vi "ORS_GalvoPrepareScan_uw-1kp.vi"(7 "SampQuant.SampMode":i32(ring)=10123 items=["Finite Samples"=10178, "Continuous Samples"=10123, "Hardware Timed Single Point"=12522], 8 "error in":errorcluster, 9 "use_digi_trig":bool, 10 "AO.DataXferMech":i32(ring)=12590 items=["DMA"=10054, "Interrupts"=10204, "Programmed I/O"=10264, "USB Bulk"=12590], 11 "Galvo":T1={"x mirror"="Dev1/ao0", "y mirror"="Dev1/ao1", "trig out"="Dev1/port0/line2", "x mirror task"="", "y mirror task"="", "trig out task"="", "n_axis"=0, "params"={"n_lines"=500, "n_frames"=400, "force to zero"=FALSE, "Triggers_per_sweep"=1.0, "X center"=0.0, "X span"=3.4000000000000004, "Y center"=0.0, "Y span"=0.0, "flyb.lines"=40, "n_triggers"=1, "mode"=3, "offset"=0.0, "galvo phase"=0, "span factor"=0.0, "Custom trig."={"n_f to c. trig"=0, "c. trig length"=0, "c. trig interval"=0, "n_c. trig"=0}, "f_per_pos"=1, "n_dataset"=1, "flyback fr"=0}, "acq trig out"="Dev1/port0/line4", "acq trig out task"="", "sample array X"=[], "sample array Y"=[], "custom trig out"="", "custom trig out task"="", "FDML-box"="TCPIP0::10.153.218.51::23::SOCKET", "ACQ/Galvo"=enum."NI_DAQ", "acq trig out an task"="", "acq trig out an"="Dev1/ao2", "Galvo Trig input"="/Dev1/PFI1", "Galvo Clk input"="OnboardClock", "sample array Acq trig out an"=[]} {"params"."n_dataset" min=1; "params"."X center" format="%^_3g"; "params"."X span" format="%^_3g"; "params"."Y center" format="%^_3g"; "params"."Y span" format="%^_3g"}) -> (0 "error out":errorcluster, 1 "# samples":i32, 2 "Galvo wfm":dbl[][](graph), 3 "Galvo out":T1={"x mirror"="Dev1/ao0", "y mirror"="Dev1/ao1", "trig out"="Dev1/port0/line2", "x mirror task"="", "y mirror task"="", "trig out task"="", "n_axis"=0, "params"={"n_lines"=500, "n_frames"=400, "force to zero"=FALSE, "Triggers_per_sweep"=1.0, "X center"=0.0, "X span"=3.4000000000000004, "Y center"=0.0, "Y span"=0.0, "flyb.lines"=40, "n_triggers"=1, "mode"=3, "offset"=0.0, "galvo phase"=0, "span factor"=0.0, "Custom trig."={"n_f to c. trig"=0, "c. trig length"=0, "c. trig interval"=0, "n_c. trig"=0}, "f_per_pos"=1, "n_dataset"=1, "flyback fr"=0}, "acq trig out"="Dev1/port0/line4", "acq trig out task"="", "sample array X"=[], "sample array Y"=[], "custom trig out"="", "custom trig out task"="", "FDML-box"="TCPIP0::10.153.218.51::23::SOCKET", "ACQ/Galvo"=enum."NI_DAQ", "acq trig out an task"="", "acq trig out an"="Dev1/ao2", "Galvo Trig input"="/Dev1/PFI1", "Galvo Clk input"="OnboardClock", "sample array Acq trig out an"=[]} {"params"."n_dataset" min=1; "params"."X center" format="%^_3g"; "params"."X span" format="%^_3g"; "params"."Y center" format="%^_3g"; "params"."Y span" format="%^_3g"})   [LabVIEW 2024]
uses:
  Typedefs/ORS_Galvo.ctl
  Typedefs/ORS_Galvo_params.ctl
  <vilib>/Utility/error.llb/DialogType.ctl
  <vilib>/DAQmx/write.llb/DAQmx Write (Digital Bool 1Line 1Point).vi
  <vilib>/DAQmx/write.llb/DAQmx Write (Analog DBL 1Chan 1Samp).vi
  <vilib>/DAQmx/write.llb/DAQmx Write (Analog 2D DBL NChan NSamp).vi
  <vilib>/DAQmx/write.llb/DAQmx Write (Analog 1D DBL NChan 1Samp).vi
  <vilib>/DAQmx/write.llb/DAQmx Write (Digital 2D U32 NChan NSamp).vi
  <vilib>/DAQmx/write.llb/DAQmx Write (Analog 1D DBL 1Chan NSamp).vi
  <vilib>/DAQmx/miscellaneous.llb/DAQmx Fill In Error Info.vi
  <resource>/objmgr/daqmx.rc
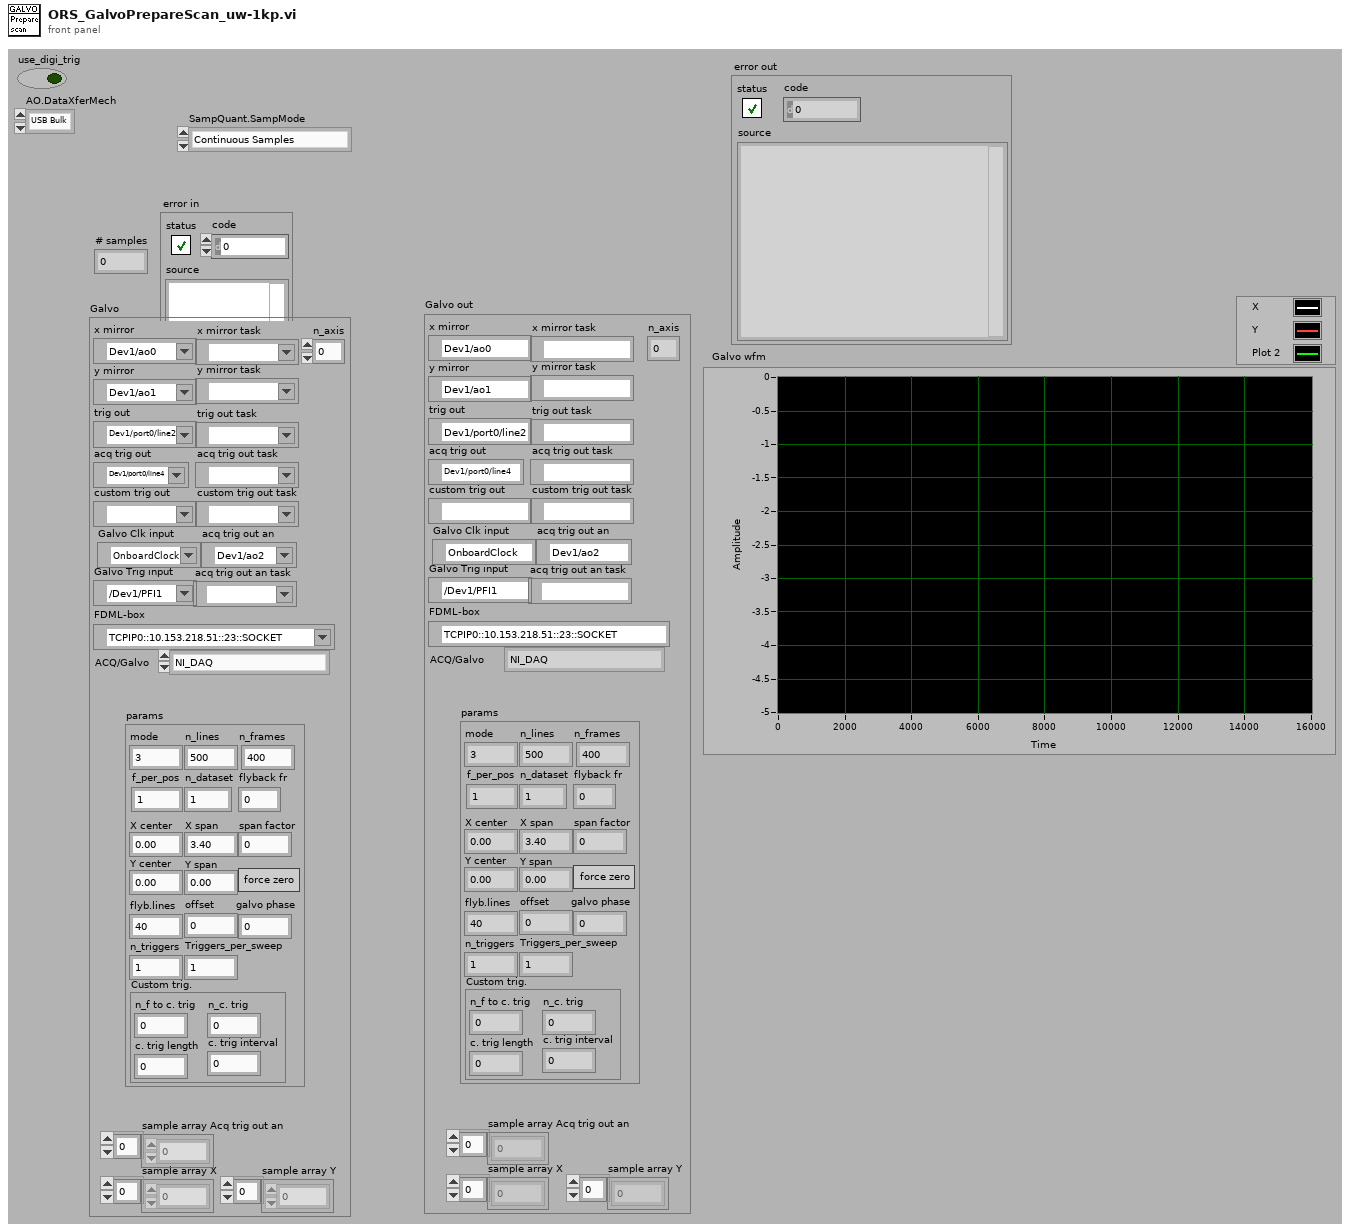
[diagram p1: front panel]
types:
  T1 = typedef "ORS_Galvo.ctl" = cluster{"x mirror":tag, "y mirror":tag, "trig out":tag, "x mirror task":refnum<k21>, "y mirror task":refnum<k21>, "trig out task":refnum<k21>, "n_axis":i32, "params":T2, "acq trig out":tag, "acq trig out task":refnum<k21>, "sample array X":dbl[], "sample array Y":dbl[], "custom trig out":tag, "custom trig out task":refnum<k21>, "FDML-box":refnum<visa-resource-name>, "ACQ/Galvo":enum16{"ADC/FDML", "NI_DAQ", "ADC"}, "acq trig out an task":refnum<k21>, "acq trig out an":tag, "Galvo Trig input":tag, "Galvo Clk input":tag, "sample array Acq trig out an":dbl[]}
  T2 = typedef "ORS_Galvo_params.ctl" = cluster{"n_lines":i32, "n_frames":i32, "force to zero":bool, "Triggers_per_sweep":dbl, "X center":dbl, "X span":dbl, "Y center":dbl, "Y span":dbl, "flyb.lines":i32, "n_triggers":i32, "mode":i32, "offset":dbl, "galvo phase":i32, "span factor":dbl, "Custom trig.":cluster{"n_f to c. trig":i32, "c. trig length":i32, "c. trig interval":i32, "n_c. trig":i32}, "f_per_pos":i32, "n_dataset":u32, "flyback fr":u16}
  T3 = typedef "DialogType.ctl" = u16
  T4 = cluster{"n_f to c. trig":i32, "c. trig length":i32, "c. trig interval":i32, "n_c. trig":i32}
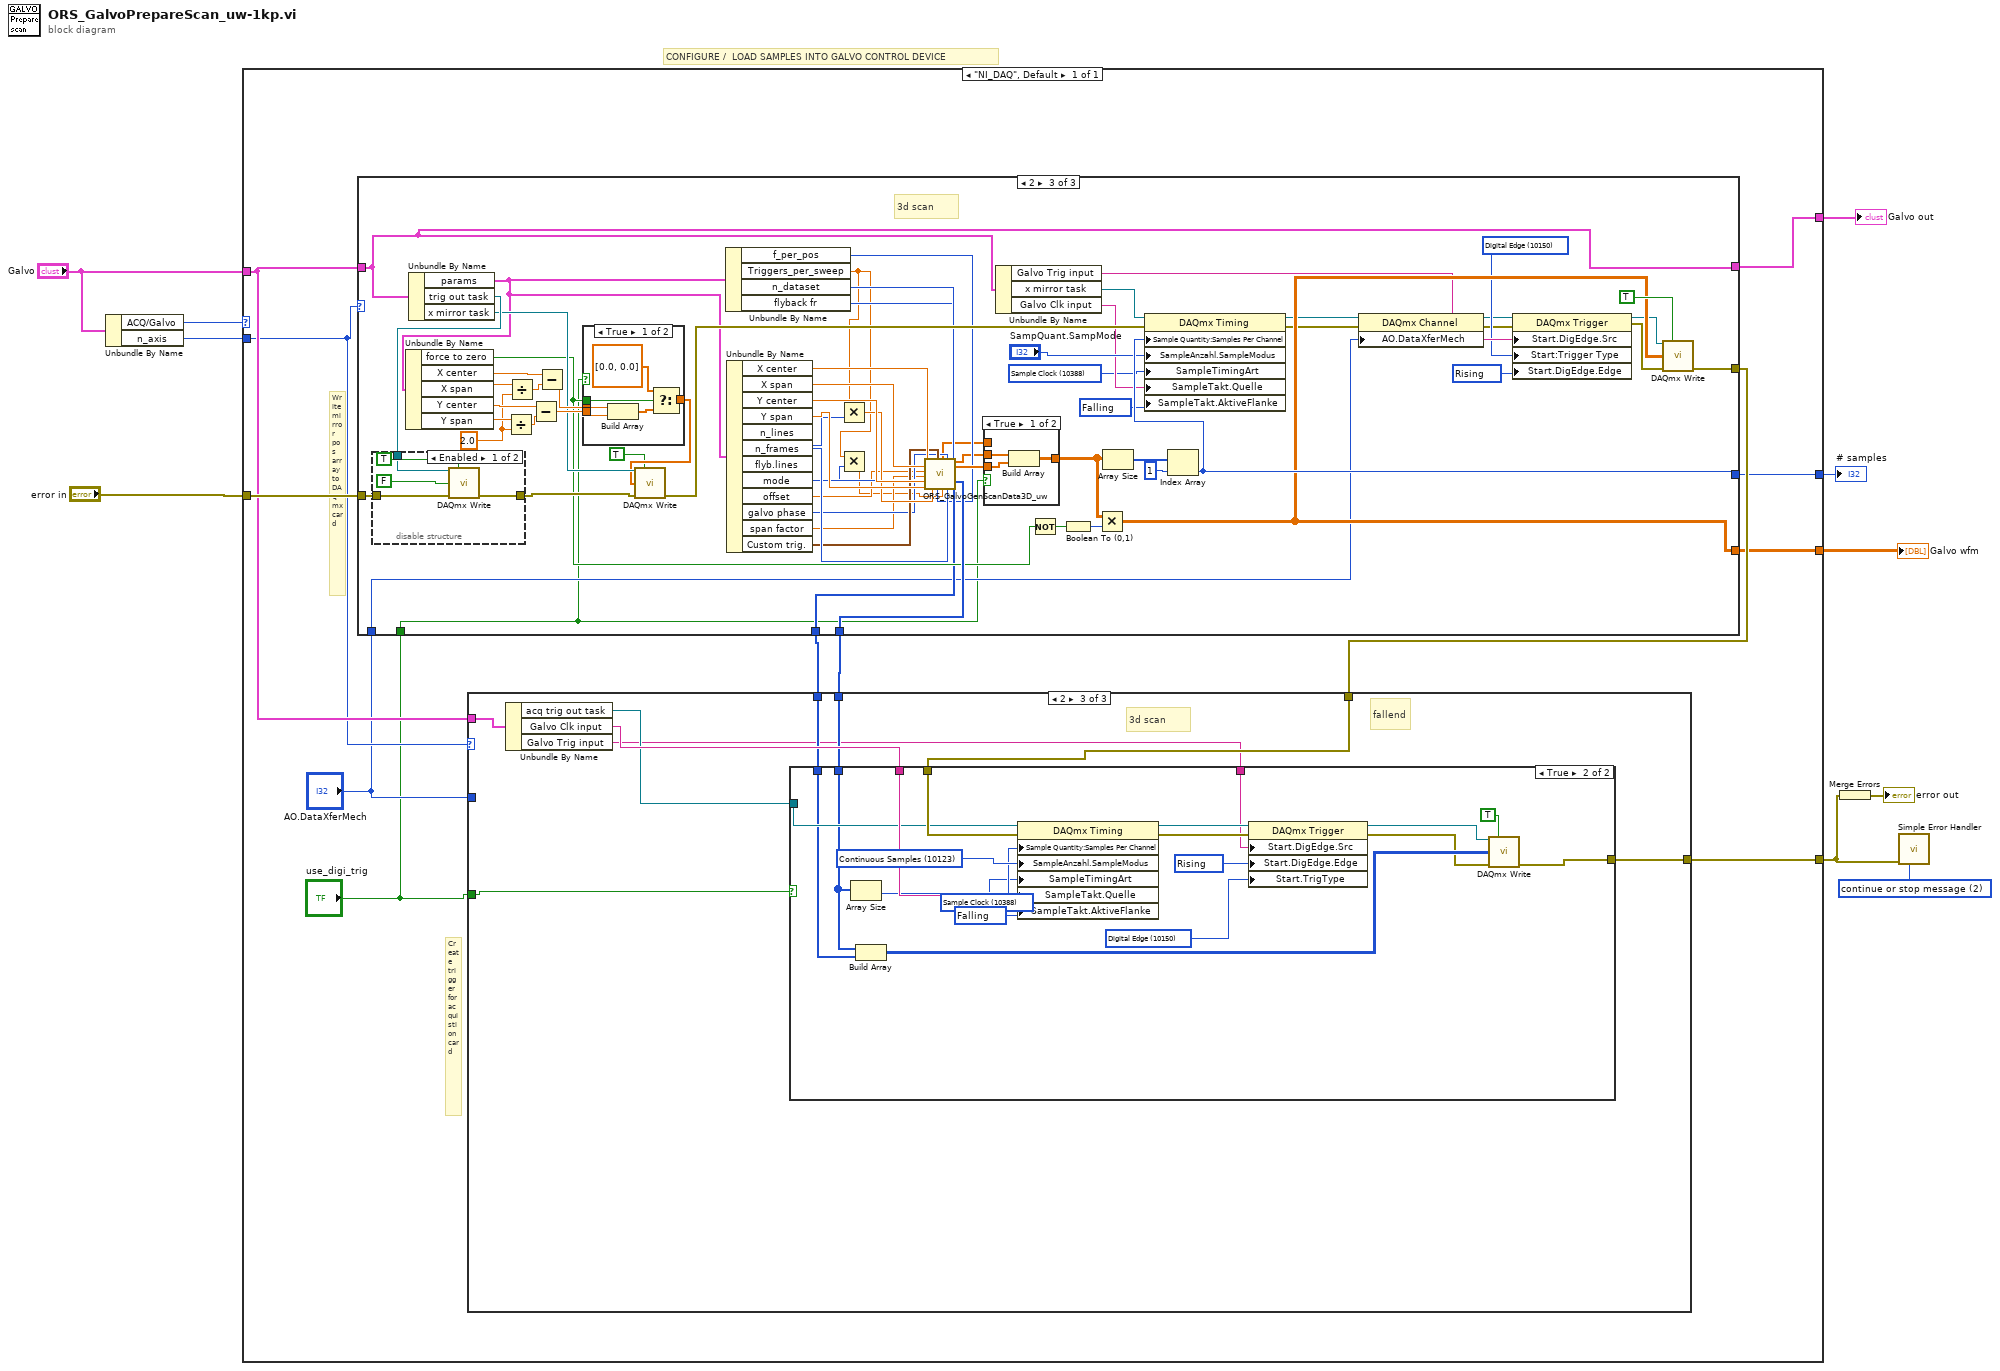
[diagram p0: block diagram]
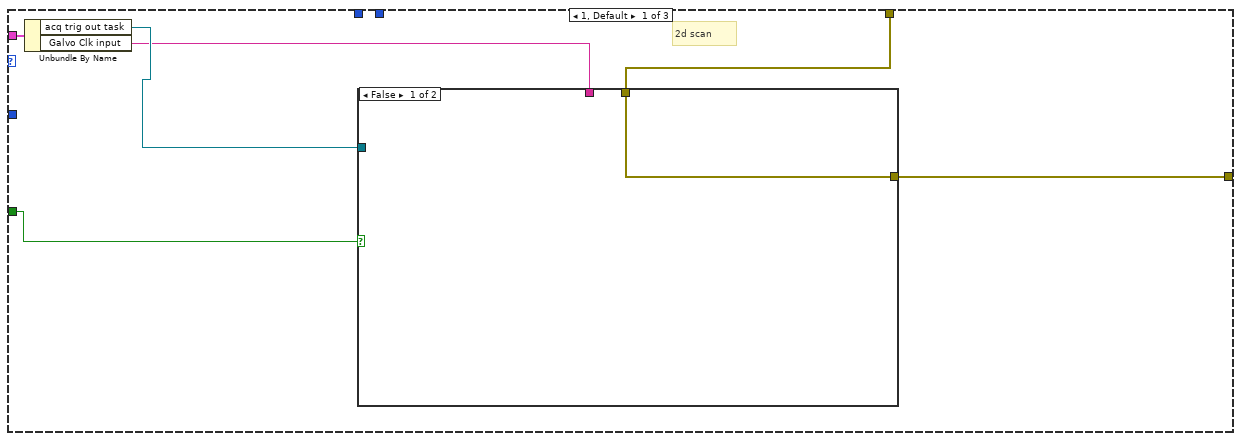
[diagram p2: hidden frame]
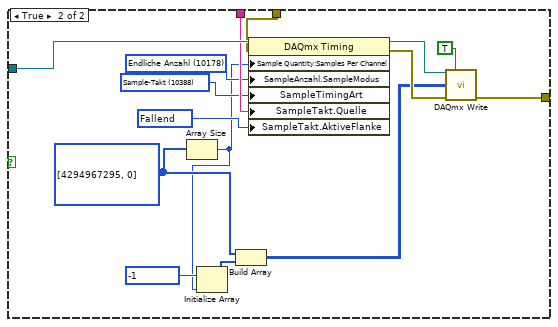
[diagram p3: hidden frame]
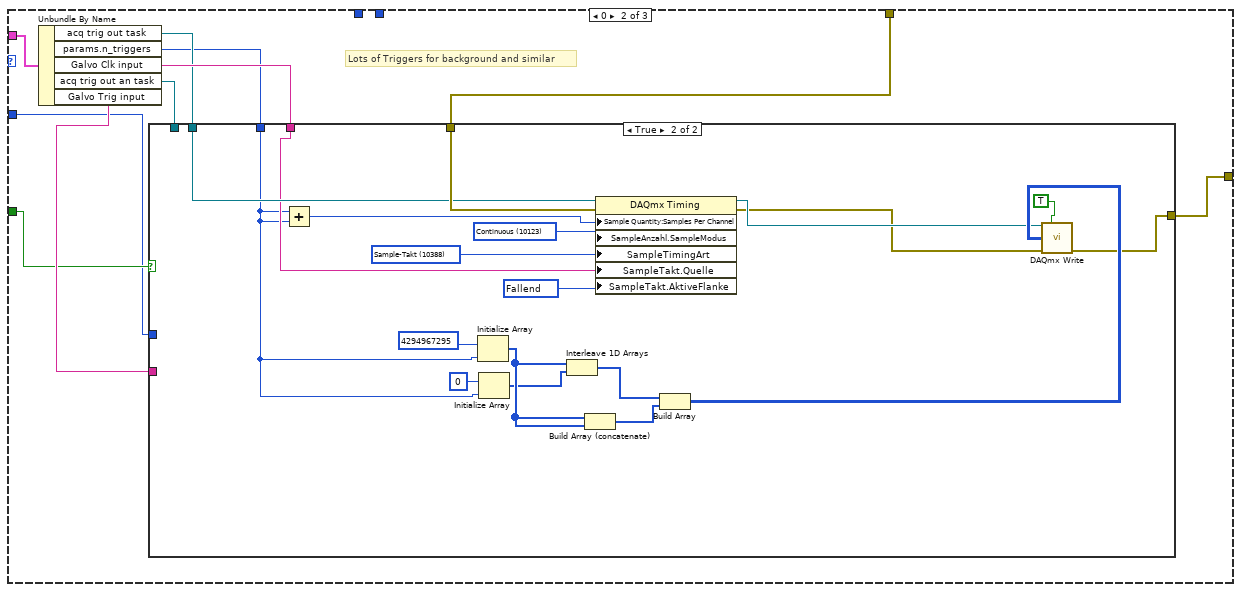
[diagram p4: hidden frame]
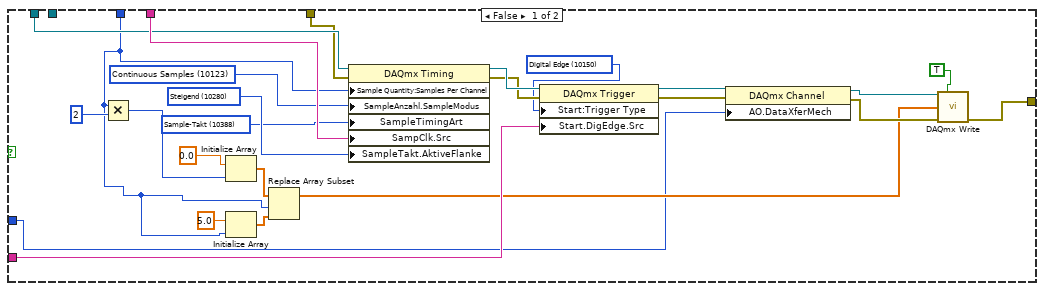
[diagram p5: hidden frame]
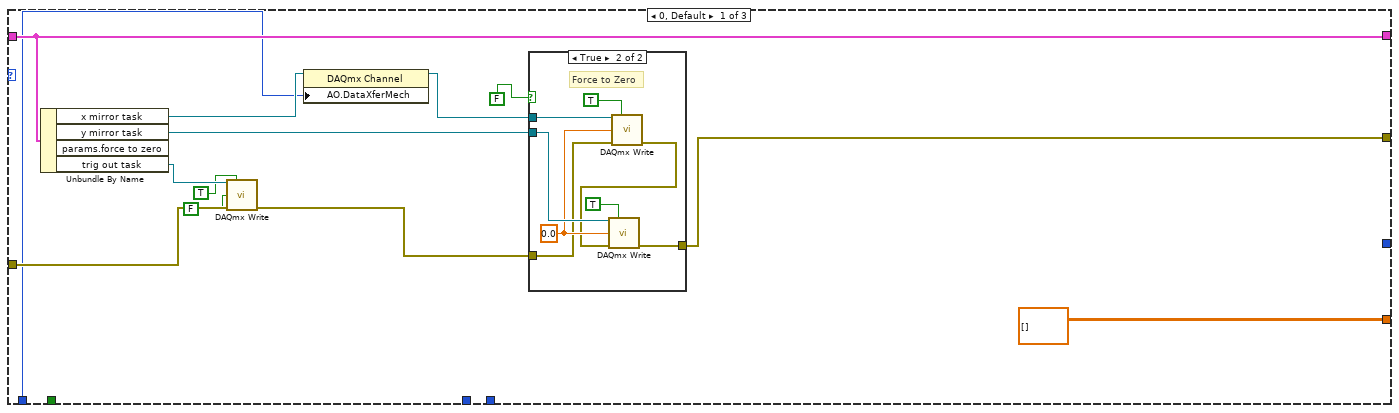
[diagram p7: hidden frame]
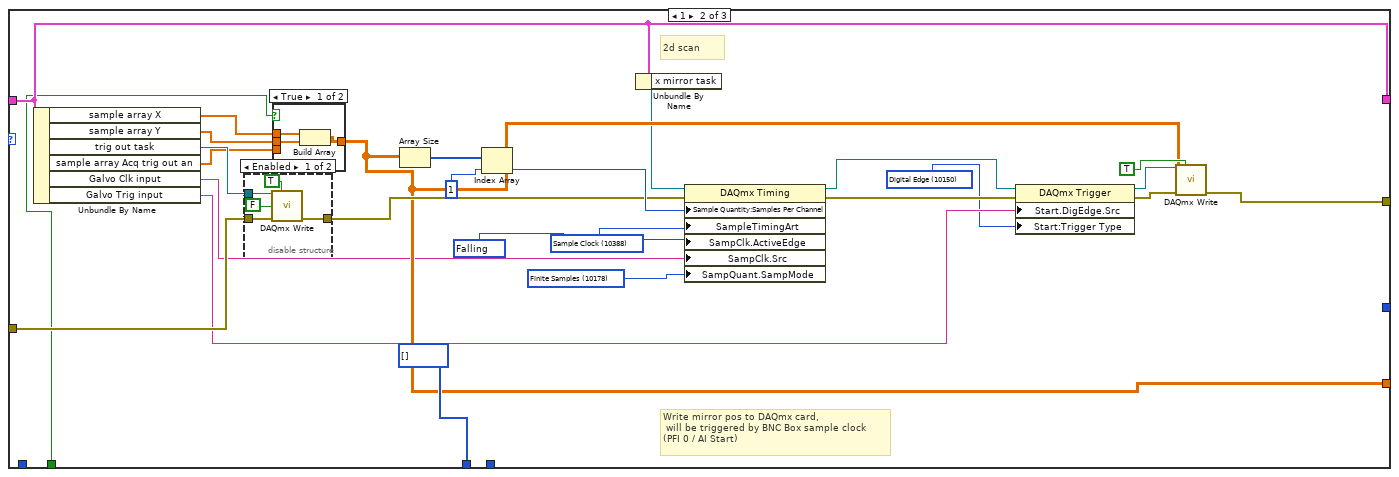
[diagram p9: hidden frame]
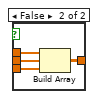
[diagram p11: hidden frame]
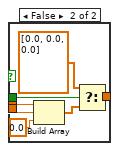
[diagram p13: hidden frame]
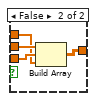
[diagram p14: hidden frame]
diagram:
  w7 = T3 2 items=["no dialog", "OK message", "continue or stop message", "OK message + warnings", "continue/stop + warnings"] ("type of dialog (OK msg:1)")
  # "CONFIGURE /  LOAD SAMPLES INTO GALVO CONTROL DEVICE"
  n1 = Unbundle By Name("Galvo") -> ("ACQ/Galvo"=w2:enum16{"ADC/FDML", "NI_DAQ", "ADC"}, "n_axis"=w1:i32)
  n2 = case shown="\"NI_DAQ\", Default" w2 {
    tunnel: "error in" -> [w22]
    tunnel: [w20] -> w8
    tunnel: [w17] -> w6
    tunnel: "Galvo" -> [w16]
    tunnel: [w15] -> w5
    tunnel: [w14] -> w4
    tunnel: w1 -> [w13]
    frame "NI_DAQ", Default {
      # "Write mirror pos array to DAQmx card"
      # "Create trigger for acquistion card"
      n3 = case shown="2" w13 {
        tunnel: w22 -> [w136 w174 w243]
        tunnel: [w139 w172 w252] -> w21
        tunnel: [w140 w161 w250] -> w17
        tunnel: w16 -> [w140 w161 w250]
        tunnel: [_ _ w244] -> w19
        tunnel: [_ u32[] [] ("custom trig out") w221] -> w18
        tunnel: [_ _ w212] -> w15
        tunnel: [dbl[][] [] w163 w206] -> w14
        tunnel: "AO.DataXferMech" -> [w128 _ w192]
        tunnel: "use_digi_trig" -> [_ w150 w191]
        frame 0, Default {
          n4 = Unbundle By Name(w140) -> ("x mirror task"=w132:refnum<k21>, "y mirror task"=w138:refnum<k21>, "trig out task"=w137:refnum<k21>)  [unwired: 1 out]
          n5 = call-poly <vilib>:"DAQmx Write.vi"("task/channels in"=w137, "auto start"=TRUE, "data"=FALSE, "error in"=w136) -> ("error out"=w135:errorcluster)  [unwired: 9 in, 2 out]
          n6 = property class="DAQmx Channel"(reference=w132, "AO.DataXferMech"=w128) -> (reference out=w131:refnum<k21>)  [unwired: 1 in, 1 out]
          n7 = case shown="True" FALSE {
            tunnel: w138 -> [_ w149]
            tunnel: w135 -> [w141 w143]
            tunnel: [w141 w147] -> w139
            tunnel: w131 -> [_ w145]
            frame False {
            }
            frame True {
              w144 = 0.0 ("t")
              # "Force to Zero"
              n8 = call-poly <vilib>:"DAQmx Write.vi"("task/channels in"=w145, "auto start"=TRUE, "data"=w144, "error in"=w143) -> ("error out"=w142:errorcluster)  [unwired: 9 in, 2 out]
              n9 = call-poly <vilib>:"DAQmx Write.vi"("task/channels in"=w149, "auto start"=TRUE, "data"=w144, "error in"=w142) -> ("error out"=w147:errorcluster)  [unwired: 9 in, 2 out]
            }
          }
        }
        frame 1 {
          w151 = 10150 items=["Analog Edge"=10099, "Digital Edge"=10150, "Digital Pattern"=10398, "Analog Window"=10103, "None"=10230] ("Start.TrigType")
          w158 = 10178 items=["Finite Samples"=10178, "Continuous Samples"=10123, "Hardware Timed Single Point"=12522] ("SampQuant.SampMode")
          w159 = 10388 items=["Sample Clock"=10388, "Burst Handshake"=12548, "Handshake"=10389, "Implicit"=10451, "On Demand"=10390, "Change Detection"=12504, "Pipelined Sample Clock"=14668] ("SampTimingType")
          w164 = 10171 items=["Rising"=10280, "Falling"=10171] ("SampClk.ActiveEdge")
          # "2d scan"
          # "Write mirror pos to DAQmx card,\n will be triggered by BNC Box sample clock\n(PFI 0 / AI Start)"
          n10 = Unbundle By Name(w161) -> ("sample array X"=w171:dbl[], "sample array Y"=w170:dbl[], "trig out task"=w175:refnum<k21>, "sample array Acq trig out an"=w162:dbl[], "Galvo Clk input"=w153:tag, "Galvo Trig input"=w154:tag)
          n11 = disable-structure shown="Enabled" {
            disable-tunnel: w175 -> [w180 _]
            disable-tunnel: w174 -> [w178 w181]
            disable-tunnel: [w176 w181] -> w166
            frame Enabled {
              n12 = call-poly <vilib>:"DAQmx Write.vi"("task/channels in"=w180, "auto start"=TRUE, "data"=FALSE, "error in"=w178) -> ("error out"=w176:errorcluster)  [unwired: 9 in, 2 out]
            }
            frame Disabled {
            }
          }
          n13 = case shown="True" w150 {
            tunnel: w171 -> [w184 w188]
            tunnel: w170 -> [w183 w187]
            tunnel: [w182 w186] -> w163
            tunnel: w162 -> [_ w185]
            frame True {
              n14 = Build Array(w184, w183) -> (w182:dbl[][])
            }
            frame False {
              n15 = Build Array(w188, w187, w185) -> (w186:dbl[][])
            }
          }
          n16 = Array Size(array=w163) -> (size(s)=w169:i32[])
          n17 = Index Array(array=w169, index=1) -> (element=w167:i32)
          n18 = Unbundle By Name(w161) -> ("x mirror task"=w160:refnum<k21>)
          n19 = property class="DAQmx Timing"(reference=w160, error in=w166, "Sample Quantity:Samples Per Channel"=w167, "SampleTimingArt"=w159, "SampClk.ActiveEdge"=w164, "SampClk.Src"=w153, "SampQuant.SampMode"=w158) -> (reference out=w152:refnum<k21>, error out=w156:errorcluster)
          n20 = property class="DAQmx Trigger"(reference=w152, error in=w156, "Start.DigEdge.Src"=w154, "Start:Trigger Type"=w151) -> (reference out=w157:refnum<k21>, error out=w155:errorcluster)
          n21 = call-poly <vilib>:"DAQmx Write.vi"("task/channels in"=w157, "auto start"=TRUE, "data"=w163, "error in"=w155) -> ("error out"=w172:errorcluster)  [unwired: 9 in, 2 out]
        }
        frame 2 {
          w189 = 10171 items=["Rising"=10280, "Falling"=10171] ("SampClk.ActiveEdge")
          w190 = 10388 items=["Sample Clock"=10388, "Burst Handshake"=12548, "Handshake"=10389, "Implicit"=10451, "On Demand"=10390, "Change Detection"=12504, "Pipelined Sample Clock"=14668] ("SampTimingType")
          w193 = 10280 items=["Rising"=10280, "Falling"=10171] ("Start.DigEdge.Edge")
          w199 = 10150 items=["Analog Edge"=10099, "Digital Edge"=10150, "Digital Pattern"=10398, "Analog Window"=10103, "None"=10230] ("Start.TrigType")
          w230 = 2.0
          # "3d scan"
          n22 = Unbundle By Name(w250) -> ("params"=w224:T2, "trig out task"=w242:refnum<k21>, "x mirror task"=w235:refnum<k21>)
          n23 = disable-structure shown="Enabled" {
            disable-tunnel: w243 -> [w258 w261]
            disable-tunnel: w242 -> [w257 _]
            disable-tunnel: [w256 w261] -> w241
            frame Enabled {
              n24 = call-poly <vilib>:"DAQmx Write.vi"("task/channels in"=w257, "auto start"=TRUE, "data"=FALSE, "error in"=w258) -> ("error out"=w256:errorcluster)  [unwired: 9 in, 2 out]
            }
            frame Disabled {
            }
          }
          n25 = Unbundle By Name(w224) -> ("force to zero"=w225:bool, "X center"=w239:dbl, "X span"=w231:dbl, "Y center"=w238:dbl, "Y span"=w234:dbl)
          n26 = Divide(x=w234, y=w230) -> (x/y=w233:dbl)
          n27 = Divide(x=w231, y=w230) -> (x/y=w232:dbl)
          n28 = Subtract(x=w238, y=w233) -> (x-y=w236:dbl)
          n29 = Subtract(x=w239, y=w232) -> (x-y=w237:dbl)
          n30 = case shown="True" w191 {
            tunnel: w237 -> [w267 w274]
            tunnel: w236 -> [w266 w273]
            tunnel: [w264 w271] -> w229
            tunnel: w225 -> [w263 w270]
            frame True {
              n31 = Build Array(w267, w266) -> (w265:dbl[])
              n32 = Select(t=dbl[] [0.0, 0.0] ("s? t:f"), s=w263, f=w265) -> (s? t:f=w264:dbl[])
            }
            frame False {
              n33 = Build Array(w274, w273, 0.0 ("element")) -> (w272:dbl[])
              n34 = Select(t=dbl[] [0.0, 0.0, 0.0] ("s? t:f"), s=w270, f=w272) -> (s? t:f=w271:dbl[])
            }
          }
          n35 = call-poly <vilib>:"DAQmx Write.vi"("task/channels in"=w235, "auto start"=TRUE, "data"=w229, "error in"=w241) -> ("error out"=w240:errorcluster)  [unwired: 9 in, 2 out]
          n36 = Unbundle By Name(w224) -> ("f_per_pos"=w215:i32, "Triggers_per_sweep"=w210:dbl, "n_dataset"=w214:u32, "flyback fr"=w213:u16)
          n37 = Unbundle By Name(w224) -> ("X center"=w249:dbl, "X span"=w248:dbl, "Y center"=w247:dbl, "Y span"=w246:dbl, "n_lines"=w223:i32, "n_frames"=w245:i32, "flyb.lines"=w209:i32, "mode"=w219:i32, "offset"=w216:dbl, "galvo phase"=w218:i32, "span factor"=w217:dbl, "Custom trig."=w220:T4)
          n38 = Multiply(x=w210, y=w223) -> (x*y=w222:dbl)
          n39 = Multiply(x=w210, y=w209) -> (x*y=w208:dbl)
          n40 = call "ORS_GalvoGenScanData3D_uw.vi"("x_center"=w249, "x_span"=w248, "offset"=w216, "span-factor"=w217, "y_center"=w247, "y_span"=w246, "mode"=w219, "n_lines"=w222, "Custom trig."=w220, "n_frames same y pos"=w215, "flyback_lines"=w208, "galvo phase"=w218, "n_frames"=w245, "n_3D scans"=w214, "flyback frames"=w213) -> ("t_data"=w205:dbl[], "x_data"=w207:dbl[], "y_data"=w251:dbl[], "trigger out"=w244:u32[], "custom trig out"=w221:u32[])
          n41 = case shown="True" w191 {
            tunnel: w251 -> [w277 w281]
            tunnel: [w276 w280] -> w228
            tunnel: w207 -> [w275 w279]
            tunnel: w205 -> [_ w278]
            frame True {
              n42 = Build Array(w275, w277) -> (w276:dbl[][])
            }
            frame False {
              n43 = Build Array(w279, w281, w278) -> (w280:dbl[][])
            }
          }
          n44 = Unbundle By Name(w250) -> ("Galvo Trig input"=w202:tag, "x mirror task"=w253:refnum<k21>, "Galvo Clk input"=w200:tag)
          n45 = Not(x=w225) -> (.not. x?=w226:bool)
          n46 = Boolean To (0,1)(Boolean=w226) -> (0, 1=w227:i16)
          n47 = Multiply(x=w228, y=w227) -> (x*y=w206:dbl[][])
          n48 = Array Size(array=w228) -> (size(s)=w211:i32[])
          n49 = Index Array(array=w211, index=1 ("Index")) -> (element=w212:i32)
          n50 = property class="DAQmx Timing"(reference=w253, error in=w240, "Sample Quantity:Samples Per Channel"=w212, "SampleAnzahl.SampleModus"="SampQuant.SampMode", "SampleTimingArt"=w190, "SampleTakt.Quelle"=w200, "SampleTakt.AktiveFlanke"=w189) -> (reference out=w198:refnum<k21>, error out=w197:errorcluster)
          n51 = property class="DAQmx Channel"(reference=w198, error in=w197, "AO.DataXferMech"=w192) -> (reference out=w196:refnum<k21>, error out=w195:errorcluster)
          n52 = property class="DAQmx Trigger"(reference=w196, error in=w195, "Start.DigEdge.Src"=w202, "Start:Trigger Type"=w199, "Start.DigEdge.Edge"=w193) -> (reference out=w204:refnum<k21>, error out=w203:errorcluster)
          n53 = call-poly <vilib>:"DAQmx Write.vi"("task/channels in"=w204, "auto start"=TRUE, "data"=w206, "error in"=w203) -> ("error out"=w252:errorcluster)  [unwired: 9 in, 2 out]
        }
      }
      n54 = case shown="2" w13 {
        tunnel: w16 -> [w28 w54 w107]
        tunnel: [w24 w53 w104] -> w20
        tunnel: w21 -> [w26 w49 w106]
        tunnel: w19 -> [_ _ w101]
        tunnel: w18 -> [_ _ w102]
        tunnel: "use_digi_trig" -> [w23 w46 w100]
        tunnel: "AO.DataXferMech" -> [_ w45 _]
        frame 1, Default {
          # "2d scan"
          n55 = Unbundle By Name(w28) -> ("acq trig out task"=w27:refnum<k21>, "Galvo Clk input"=w25:tag)
          n56 = case shown="False" w23 {
            tunnel: w27 -> [_ w44]
            tunnel: w26 -> [w29 w43]
            tunnel: w25 -> [_ w42]
            tunnel: [w29 w41] -> w24
            frame False {
            }
            frame True {
              w34 = u32[] [4294967295, 0] ("data")
              w38 = 10171 items=["Steigend"=10280, "Fallend"=10171] ("SampleTakt.AktiveFlanke")
              w39 = 10178 items=["Endliche Anzahl"=10178, "kontinuierlich"=10123, "Einzelwert (HW-getaktet)"=12522] ("SampleAnzahl.SampleModus")
              w40 = 10388 items=["Sample-Takt"=10388, "Burst-Handshake"=12548, "Handshake"=10389, "implizit"=10451, "1 Sample"=10390, "Änderungserkennung"=12504, "Sample-Takt in Pipeline"=14668] ("SampleTimingArt")
              n57 = Array Size(array=w34) -> (size(s)=w31:i32)
              n58 = Initialize Array(-1 ("Waveform"), w31) -> (w30:i32[])
              n59 = Build Array(w34, w30) -> (w33:u32[][])
              n60 = property class="DAQmx Timing"(reference=w44, error in=w43, "Sample Quantity:Samples Per Channel"=w31, "SampleAnzahl.SampleModus"=w39, "SampleTimingArt"=w40, "SampleTakt.Quelle"=w42, "SampleTakt.AktiveFlanke"=w38) -> (reference out=w37:refnum<k21>, error out=w36:errorcluster)
              n61 = call-poly <vilib>:"DAQmx Write.vi"("task/channels in"=w37, "auto start"=TRUE, "data"=w33, "error in"=w36) -> ("error out"=w41:errorcluster)  [unwired: 9 in, 2 out]
            }
          }
        }
        frame 0 {
          # "Lots of Triggers for background and similar"
          n62 = Unbundle By Name(w54) -> ("acq trig out task"=w48:refnum<k21>, "params.n_triggers"=w47:i32, "Galvo Clk input"=w52:tag, "acq trig out an task"=w51:refnum<k21>, "Galvo Trig input"=w50:tag)
          n63 = case shown="True" w46 {
            tunnel: [w79 w84] -> w53
            tunnel: w52 -> [w78 w83]
            tunnel: w51 -> [w77 _]
            tunnel: w50 -> [w76 _]
            tunnel: w49 -> [w59 w86]
            tunnel: w48 -> [_ w85]
            tunnel: w47 -> [w56 w82]
            tunnel: w45 -> [w55 _]
            frame False {
              w60 = 10150 items=["Analog Edge"=10099, "Digital Edge"=10150, "Digital Pattern"=10398, "Analog Window"=10103, "None"=10230] ("Start.TrigType")
              w69 = 10123 items=["Finite Samples"=10178, "Continuous Samples"=10123, "Hardware Timed Single Point"=12522] ("SampQuant.SampMode")
              w73 = 10280 items=["Steigend"=10280, "Fallend"=10171] ("SampleTakt.AktiveFlanke")
              w72 = 10388 items=["Sample-Takt"=10388, "Burst-Handshake"=12548, "Handshake"=10389, "implizit"=10451, "1 Sample"=10390, "Änderungserkennung"=12504, "Sample-Takt in Pipeline"=14668] ("SampleTimingArt")
              n64 = Multiply(x=w56, y=2) -> (x*y=w57:i32)
              n65 = Initialize Array(0.0, w57) -> (w63:dbl[])
              n66 = Initialize Array(5.0, w56) -> (w62:dbl[])
              n67 = Replace Array Subset(array=w63, new element=w62, index=w56) -> (w61:dbl[])
              n68 = property class="DAQmx Timing"(reference=w77, error in=w59, "Sample Quantity:Samples Per Channel"=w56, "SampleAnzahl.SampleModus"=w69, "SampleTimingArt"=w72, "SampClk.Src"=w78, "SampleTakt.AktiveFlanke"=w73) -> (reference out=w71:refnum<k21>, error out=w70:errorcluster)
              n69 = property class="DAQmx Trigger"(reference=w71, error in=w70, "Start:Trigger Type"=w60, "Start.DigEdge.Src"=w76) -> (reference out=w68:refnum<k21>, error out=w67:errorcluster)
              n70 = property class="DAQmx Channel"(reference=w68, error in=w67, "AO.DataXferMech"=w55) -> (reference out=w66:refnum<k21>, error out=w65:errorcluster)
              n71 = call-poly <vilib>:"DAQmx Write.vi"("task/channels in"=w66, "auto start"=TRUE, "data"=w61, "error in"=w65) -> ("error out"=w79:errorcluster)  [unwired: 9 in, 2 out]
            }
            frame True {
              w89 = 10171 items=["Steigend"=10280, "Fallend"=10171] ("SampleTakt.AktiveFlanke")
              w88 = 10123 items=["Finite samplies"=10178, "Continuous"=10123, "Einzelwert (HW-getaktet)"=12522] ("SampleAnzahl.SampleModus")
              w87 = 10388 items=["Sample-Takt"=10388, "Burst-Handshake"=12548, "Handshake"=10389, "implizit"=10451, "1 Sample"=10390, "Änderungserkennung"=12504, "Sample-Takt in Pipeline"=14668] ("SampleTimingArt")
              n72 = Add(x=w82, y=w82) -> (x+y=w97:i32)
              n73 = Initialize Array(u32 4294967295 ("Waveform"), w82) -> (w98:u32[])
              n74 = Initialize Array(u32 0 ("Waveform"), w82) -> (w94:u32[])
              n75 = Interleave 1D Arrays(w98, w94) -> (w93:u32[])
              n76 = Build Array (concatenate)(w98, w98) -> (w95:u32[])
              n77 = property class="DAQmx Timing"(reference=w85, error in=w86, "Sample Quantity:Samples Per Channel"=w97, "SampleAnzahl.SampleModus"=w88, "SampleTimingArt"=w87, "SampleTakt.Quelle"=w83, "SampleTakt.AktiveFlanke"=w89) -> (reference out=w81:refnum<k21>, error out=w80:errorcluster)
              n78 = Build Array(w93, w95) -> (w96:u32[][])
              n79 = call-poly <vilib>:"DAQmx Write.vi"("task/channels in"=w81, "auto start"=TRUE, "data"=w96, "error in"=w80) -> ("error out"=w84:errorcluster)  [unwired: 9 in, 2 out]
            }
          }
        }
        frame 2 {
          # "fallend"
          # "3d scan"
          n80 = Unbundle By Name(w107) -> ("acq trig out task"=w103:refnum<k21>, "Galvo Clk input"=w105:tag, "Galvo Trig input"=w99:tag)
          n81 = case shown="True" w100 {
            tunnel: w106 -> [w108 w127]
            tunnel: w105 -> [_ w126]
            tunnel: [w108 w125] -> w104
            tunnel: w103 -> [_ w124]
            tunnel: w102 -> [_ w123]
            tunnel: w101 -> [_ w122]
            tunnel: w99 -> [_ w113]
            frame False {
            }
            frame True {
              w109 = 10171 items=["Rising"=10280, "Falling"=10171] ("SampClk.ActiveEdge")
              w110 = 10388 items=["Sample Clock"=10388, "Burst Handshake"=12548, "Handshake"=10389, "Implicit"=10451, "On Demand"=10390, "Change Detection"=12504, "Pipelined Sample Clock"=14668] ("SampTimingType")
              w121 = 10123 items=["Finite Samples"=10178, "Continuous Samples"=10123, "Hardware Timed Single Point"=12522] ("SampQuant.SampMode")
              w111 = 10150 items=["Analog Edge"=10099, "Digital Edge"=10150, "Digital Pattern"=10398, "Analog Window"=10103, "None"=10230] ("Start.TrigType")
              w112 = 10280 items=["Rising"=10280, "Falling"=10171] ("Start.DigEdge.Edge")
              n82 = Array Size(array=w122) -> (size(s)=w118:i32)
              n83 = Build Array(w122, w123) -> (w119:u32[][])
              n84 = property class="DAQmx Timing"(reference=w124, error in=w127, "Sample Quantity:Samples Per Channel"=w118, "SampleAnzahl.SampleModus"=w121, "SampleTimingArt"=w110, "SampleTakt.Quelle"=w126, "SampleTakt.AktiveFlanke"=w109) -> (reference out=w115:refnum<k21>, error out=w116:errorcluster)
              n85 = property class="DAQmx Trigger"(reference=w115, error in=w116, "Start.DigEdge.Src"=w113, "Start.DigEdge.Edge"=w112, "Start.TrigType"=w111) -> (reference out=w114:refnum<k21>, error out=w117:errorcluster)
              n86 = call-poly <vilib>:"DAQmx Write.vi"("task/channels in"=w114, "auto start"=TRUE, "data"=w119, "error in"=w117) -> ("error out"=w125:errorcluster)  [unwired: 9 in, 2 out]
            }
          }
        }
      }
    }
  }
  "Galvo out" <- w6
  "# samples" <- w5
  "Galvo wfm" <- w4
  n87 = Merge Errors(w8) -> (→"error out":errorcluster)
  n88 = call <vilib>:"Simple Error Handler.vi"("type of dialog (OK msg:1)"=w7, "error in (no error)"=w8) -> ()  [unwired: 3 in, 5 out]
